vi "编码器测量实验.vi"   [LabVIEW 2011]
uses:
  <vilib>/STM32_DriverVI_Interface_F4/Timer/TIM5_Group_Pins_F4.ctl
  <vilib>/STM32_DriverVI_Interface_F4/Timer/TIM5_Channels_Pin_Map_F4.ctl
  <vilib>/STM32_DriverVI_Interface_F4/GPIO/GPIO_Group_Mode_Interface_F4.ctl
  <vilib>/STM32_DriverVI_Interface_F4/Timer/Filter Mode_F4.ctl
  <vilib>/STM32_DriverVI_Interface_F4/Timer/TIM5_Capture_Channel_F4.ctl
  <vilib>/STM32_DriverVI_Interface_F4/Timer/Edge Mode_F4.ctl
  <vilib>/STM32_DriverVI_Interface_F4/Timer/TIMX Interrupt_F4.ctl
  <vilib>/STM32_DriverVI_Interface_F4/Interrupt/PreemptionPriority_2_F4.ctl
  <vilib>/STM32_DriverVI_Interface_F4/Interrupt/SubPriority_2_F4.ctl
  <vilib>/STM32_DriverVI_Interface_F4/Timer/TIM5_Int_Channel_F4.ctl
  <vilib>/STM32_DriverVI_Interface_F4/LCD/Show_Mode_F4.ctl
  <vilib>/STM32_DriverVI_Interface_F4/LCD/Font_Size_F4.ctl
  <vilib>/STM32_DriverVI_Interface_F4/LCD/Brush Color_Index_F4.ctl
  <vilib>/STM32_DriverVI_Interface_F4/LCD/LCD_Init_F4.vi
  <vilib>/STM32_DriverVI_Interface_F4/Timer/TIM5 Init_F4.vi
  <vilib>/STM32_DriverVI_Interface_F4/Timer/TIM5 Channel Pin Map_F4.vi
  <vilib>/STM32_DriverVI_Interface_F4/Timer/TIM5 Channel Filter Set_F4.vi
  <vilib>/STM32_DriverVI_Interface_F4/Timer/TIM5 Channel Edge Set_F4.vi
  <vilib>/STM32_DriverVI_Interface_F4/Timer/TIM5 Encoder Mode Set_F4.vi
  <vilib>/STM32_DriverVI_Interface_F4/Timer/TIM Priority Set_2_F4.vi
  <vilib>/STM32_DriverVI_Interface_F4/Timer/TIM5 Int Permit_UnPermit_F4.vi
  <vilib>/STM32_DriverVI_Interface_F4/Timer/TIM5 Int Enable_Disable_F4.vi
  <vilib>/STM32_DriverVI_Interface_F4/Timer/TIM5 Encoder Get CNT_F4.vi
  <vilib>/STM32_DriverVI_Interface_F4/Timer/TIM5 SW Interrupt_F4.vi
  <vilib>/STM32_DriverVI_Interface_F4/Timer/Clear_TIM5_Flag_F4.vi
  <vilib>/STM32_DriverVI_Interface_F4/Timer/TIM5_Flag_F4.ctl
types:
  T1 = typedef "中断使能禁止.ctl" = enum8{"Disable", "Enable"}
  T2 = typedef "允许或禁止TIM中断_F4.ctl" = enum8{"禁止", "允许"}
  T3 = typedef "TIM5_Int_Channel_F4.ctl" = enum8{"TIM5_Update(Overflow)", "TIM5_Channel_1", "TIM5_Channel_2", "TIM5_Channel_3", "TIM5_Channel_4", "TIM5_Reserved……", "TIM5_Trigger(Pulse)"}
  T4 = typedef "SubPriority_2_F4.ctl" = enum8{"Priority_0（High）", "Priority_1", "Priority_2", "Priority_3（Low）"}
  T5 = typedef "PreemptionPriority_2_F4.ctl" = enum8{"Priority_0（Highest）", "Priority_1", "Priority_2", "Priority_3（Lowest）"}
  T6 = typedef "TIMX Interrupt_F4.ctl" = u8
  T7 = typedef "Edge Mode_F4.ctl" = enum8{"Rising edge", "Falling edge"}
  T8 = typedef "TIM5_Capture_Channel_F4.ctl" = enum8{"TIM5_Channel_1", "TIM5_Channel_2", "TIM5_Channel_3", "TIM5_Channel_4"}
  T9 = typedef "Filter Mode_F4.ctl" = enum8{"None Filter", "2 Points Filter", "4 Points Filter", "8 Points Filter"}
  T10 = typedef "GPIO_Group_Mode_Interface_F4.ctl" = enum8{"Floating Input", "Pull-up Input", "Pull-down Input", "-----------------------", "Push-pull Output", "Open-drain Output"}[]
  T11 = typedef "TIM5_Group_Pins_F4.ctl" = T12[]
  T12 = typedef "TIM5_Channels_Pin_Map_F4.ctl" = enum8{"TIM5_Channel_1-->PA0", "TIM5_Channel_1-->PH10", "TIM5_Channel_2-->PA1", "TIM5_Channel_2-->PH11", "TIM5_Channel_3-->PA2", "TIM5_Channel_3-->PH12", "TIM5_Channel_4-->PA3", "TIM5_Channel_4-->PI0"}
  T13 = typedef "TIMX计数时钟频率_F4.ctl" = u16
  T14 = typedef "TIM5_Flag_F4.ctl" = enum8{"TIM5_Update(Overflow)", "TIM5_Channel_1", "TIM5_Channel_2", "TIM5_Channel_3", "TIM5_Channel_4", "TIM5_Reserved……", "TIM5_Trigger(Pulse)"}
  T15 = typedef "Show_Mode_F4.ctl" = enum8{"非叠加显示", "叠加显示"}
  T16 = typedef "Font_Size_F4.ctl" = enum8{"Small_Font（12）", "Big_Font（16）"}
  T17 = typedef "Brush Color_Index_F4.ctl" = enum8{"White", "Black", "Blue", "Green_Blue", "Red", "Magenta（品红）", "Green", "Cyan（青色）", "Yellow", "Brown", "Brown_Red", "Gray", "Dark_Blue", "Light_Blue", "Gray_Blue", "Light_Green", "Light_Gray", "Light_Gray_Blue", "Light_Brown_Blue"}
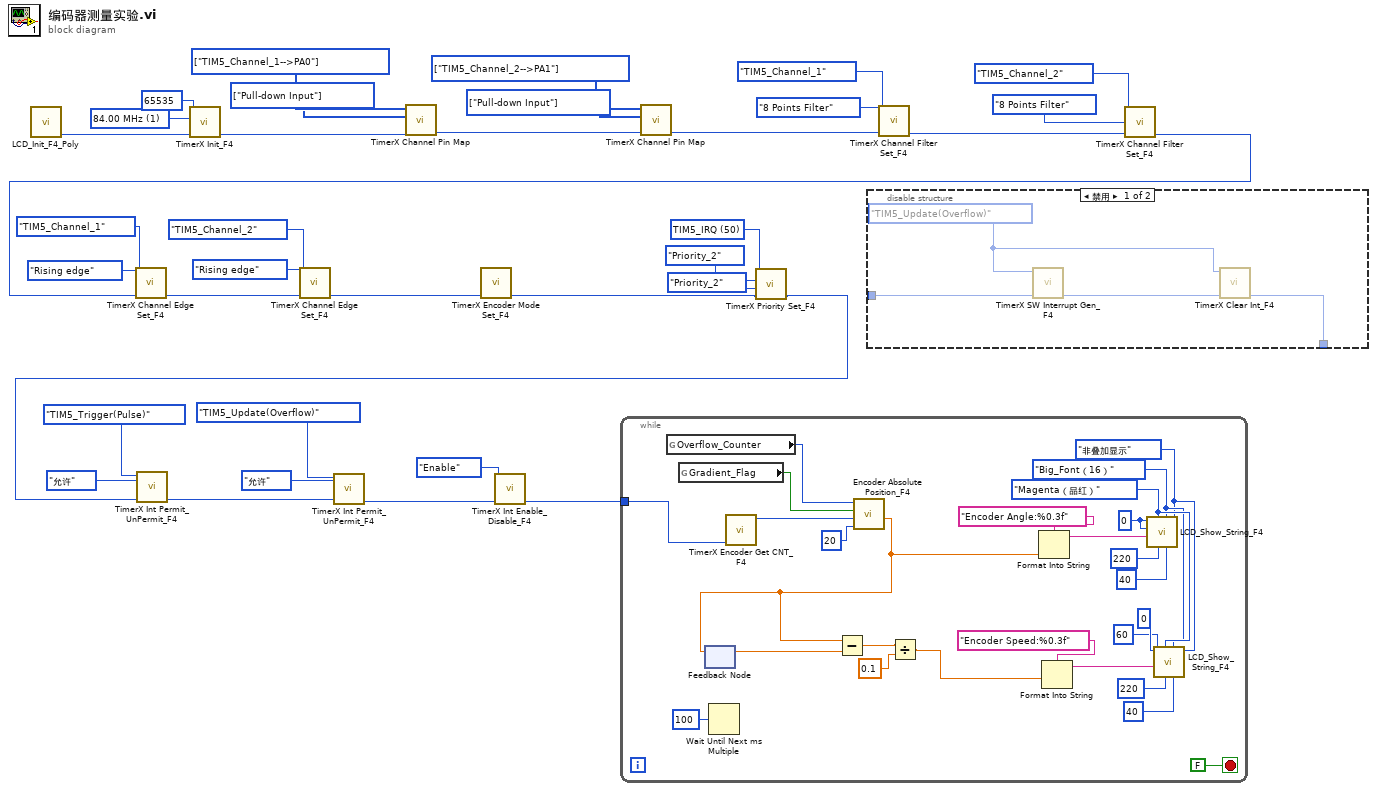
[diagram p0: block diagram]
diagram:
  w10 = T6 50 items=["WWDG_IRQ"=0, "RTC_WKUP_IRQ"=3, "RTC_Alarm_IRQ"=41, "TIM1_BRK_TIM9_IRQ"=24, "TIM1_UP_TIM10_IRQ"=25, "TIM1_TRG_COM_TIM11_IRQ"=26, "TIM1_CC_IRQ"=27, "TIM2_IRQ"=28, "TIM3_IRQ"=29, "TIM4_IRQ"=30, "TIM5_IRQ"=50, "TIM6_IRQ"=54, "TIM7_IRQ"=55, "TIM8_BRK_TIM12_IRQ"=43, "TIM8_UP_TIM13_IRQ"=44, "TIM8_TRG_COM_TIM14_IRQ"=45, "TIM8_CC_IRQ"=46] ("TIM 中断号设置")
  w25 = T10 [enum."Pull-down Input"] items=["Floating Input", "Pull-up Input", "Pull-down Input", "-----------------------", "Push-pull Output", "Open-drain Output"] ("GPIO Mode Set")
  w26 = T11 [enum."TIM5_Channel_2-->PA1"] items=["TIM5_Channel_1-->PA0", "TIM5_Channel_1-->PH10", "TIM5_Channel_2-->PA1", "TIM5_Channel_2-->PH11", "TIM5_Channel_3-->PA2", "TIM5_Channel_3-->PH12", "TIM5_Channel_4-->PA3", "TIM5_Channel_4-->PI0"] ("TIM5 Group Channel Pins")
  w27 = T10 [enum."Pull-down Input"] items=["Floating Input", "Pull-up Input", "Pull-down Input", "-----------------------", "Push-pull Output", "Open-drain Output"] ("GPIO Mode Set")
  w28 = T11 [enum."TIM5_Channel_1-->PA0"] items=["TIM5_Channel_1-->PA0", "TIM5_Channel_1-->PH10", "TIM5_Channel_2-->PA1", "TIM5_Channel_2-->PH11", "TIM5_Channel_3-->PA2", "TIM5_Channel_3-->PH12", "TIM5_Channel_4-->PA3", "TIM5_Channel_4-->PI0"] ("TIM5 Group Channel Pins")
  w34 = T13 1 items=["84.00 MHz"=1, "42.00 MHz"=2, "28.00 MHz"=3, "21.00 MHz"=4, "12.000 MHz"=7, "7.000 MHz"=12, "4.000 MHz"=21, "1.000 MHz"=84, "-------------"=0, "500.0 KHz"=168, "250.0 KHz"=336, "100.0 KHz"=840, "50.00 KHz"=1680, "10.00 KHz"=8400] ("时钟预分频数")
  n1 = call-poly <vilib>:"LCD_Init_F4_Poly.vi"() -> ("err_out"=w33:u8)  [unwired: 10 in, 1 out]
  n2 = call-poly <vilib>:"TimerX Init_F4.vi"("err_in"=w33, "时钟预分频数"=w34, "自动重装值"=u16 65535) -> ("err_out"=w32:u8)  [unwired: 8 in]
  n3 = call-poly <vilib>:"TimerX Channel Pin Map.vi"("err_in"=w32, "GPIO Mode Set"=w27, "TIM5 Group Channel Pins"=w28) -> ("err_out"=w31:u8)  [unwired: 8 in]
  n4 = call-poly <vilib>:"TimerX Channel Pin Map.vi"("err_in"=w31, "GPIO Mode Set"=w25, "TIM5 Group Channel Pins"=w26) -> ("err_out"=w30:u8)  [unwired: 8 in]
  n5 = disable-structure shown="禁用" {
    disable-tunnel: [w38 _] -> _
    disable-tunnel: _ -> [w37 _]
    frame Disabled {
      w36 = TIM5_Flag_F4."TIM5_Update(Overflow)" ("TIM5_Flag")
      n6 = call-poly <vilib>:"TimerX SW Interrupt Gen_F4.vi"("err_in"=w37, "TIM5_Flag"=w36) -> ("err_out"=w39:u8)  [unwired: 9 in]
      n7 = call-poly <vilib>:"TimerX Clear Int_F4.vi"("err_in"=w39, "TIM5_Flag"=w36) -> ("err_out"=w38:u8)  [unwired: 9 in]
    }
    frame Enabled {
    }
  }
  n8 = call-poly <vilib>:"TimerX Channel Filter Set_F4.vi"("err_in"=w30, "Filter Mode"=Filter_Mode_F4."8 Points Filter", "TIM5_Capture_Channel"=TIM5_Capture_Channel_F4."TIM5_Channel_1") -> ("err_out"=w29:u8)  [unwired: 8 in]
  n9 = call-poly <vilib>:"TimerX Channel Filter Set_F4.vi"("err_in"=w29, "Filter Mode"=Filter_Mode_F4."8 Points Filter", "TIM5_Capture_Channel"=TIM5_Capture_Channel_F4."TIM5_Channel_2") -> ("err_out"=w20:u8)  [unwired: 8 in]
  n10 = call-poly <vilib>:"TimerX Channel Edge Set_F4.vi"("err_in"=w20, "Edge Mode"=Edge_Mode_F4."Rising edge", "TIM5_Capture_Channel"=TIM5_Capture_Channel_F4."TIM5_Channel_1") -> ("err_out"=w19:u8)  [unwired: 8 in]
  n11 = call-poly <vilib>:"TimerX Channel Edge Set_F4.vi"("err_in"=w19, "Edge Mode"=Edge_Mode_F4."Rising edge", "TIM5_Capture_Channel"=TIM5_Capture_Channel_F4."TIM5_Channel_2") -> ("err_out"=w18:u8)  [unwired: 8 in]
  n12 = call-poly <vilib>:"TimerX Encoder Mode Set_F4.vi"("err_in"=w18) -> ("err_out"=w11:u8)  [unwired: 10 in]
  n13 = call-poly <vilib>:"TimerX Priority Set_F4.vi"("err_in"=w11, "响应优先级"=SubPriority_2_F4."Priority_2", "抢占优先级"=PreemptionPriority_2_F4."Priority_2", "IO 中断号设置"=w10) -> ("err_out"=w1:u8)  [unwired: 6 in, 1 out]
  n14 = call-poly <vilib>:"TimerX Int Permit_UnPermit_F4.vi"("err_in"=w1, "屏蔽或开启TIM4中断"=允许或禁止TIM中断_F4."允许", "TIM5_Int_Channel"=TIM5_Int_Channel_F4."TIM5_Trigger(Pulse)") -> ("err_out"=w17:u8)  [unwired: 8 in]
  n15 = call-poly <vilib>:"TimerX Int Permit_UnPermit_F4.vi"("err_in"=w17, "屏蔽或开启TIM4中断"=允许或禁止TIM中断_F4."允许", "TIM5_Int_Channel"=TIM5_Int_Channel_F4."TIM5_Update(Overflow)") -> ("err_out"=w16:u8)  [unwired: 8 in]
  n16 = call-poly <vilib>:"TimerX Int Enable_Disable_F4.vi"("err_in"=w16, "中断使能/关闭"=中断使能禁止."Enable") -> ("err_out"=w2:u8)  [unwired: 9 in]
  n17 = while {
    tunnel: w2 -> [w64]
    stop <- FALSE stop-if-true
    w51 = Show_Mode_F4."非叠加显示" ("Show_Mode")
    w52 = Font_Size_F4."Big_Font（16）" ("Font_Size")
    w53 = Brush_Color_Index_F4."Magenta（品红）" ("Brush Color")
    w58 = u16 0 ("X_Position")
    n18 = global read "全局变量.vi" "Overflow_Counter"() -> (w63:u16)
    n19 = global read "全局变量.vi" "Gradient_Flag"() -> (w62:bool)
    n20 = feedback #1() -> (w42:dbl)  [unwired: 1 in]
    n21 = Wait Until Next ms Multiple(millisecond multiple=u32 100 ("毫秒倍数")) -> ()  [unwired: 1 out]
    n22 = call-poly <vilib>:"TimerX Encoder Get CNT_F4.vi"("err_in"=w64) -> ("Counter_Value"=w61:u16)  [unwired: 8 in, 2 out]
    n23 = call <vilib>:"Encoder Absolute Position_F4.vi"("Encoder_Lines/Rev"=u16 20, "Counter_Value"=w61, "Gradient_Flag"=w62, "Overflow_Counter"=w63) -> ("Absolute_Position（°）"=w43:dbl)  [unwired: 6 in, 1 out]
    n24 = feedback-in #1(w43) -> ()
    n25 = Subtract(x=w43, y=w42) -> (x-y=w44:dbl)
    n26 = Divide(x=w44, y=0.1) -> (x/y=w45:dbl)
    n27 = Format Into String(format string="Encoder Angle:%0.3f" ("初始字符串"), w43) -> (resulting string=w48:string)  [unwired: 2 in, 1 out]
    n28 = Format Into String(format string="Encoder Speed:%0.3f" ("初始字符串"), w45) -> (resulting string=w47:string)  [unwired: 2 in, 1 out]
    n29 = call <vilib>:"LCD_Show_String_F4.vi"("Show_Mode"=w51, "Height"=u16 40, "Font_Size"=w52, "Width"=u16 220, "Brush Color"=w53, "String"=w48, "Y_Position"=w58, "X_Position"=w58) -> ()  [unwired: 3 in, 1 out]
    n30 = call <vilib>:"LCD_Show_String_F4.vi"("Show_Mode"=w51, "Height"=u16 40, "Font_Size"=w52, "Width"=u16 220, "Brush Color"=w53, "String"=w47, "Y_Position"=u16 60, "X_Position"=u16 0) -> ()  [unwired: 3 in, 1 out]
  }
